vi "Set Value.vi"(8 "error in (no error)":errorcluster, 10 "Value":variant, 11 "IAttribute Data Type View in":refnum<class "IAttribute Data Type View.lvclass">) -> (0 "error out":errorcluster, 3 "IAttribute Data Type View out":refnum<class "IAttribute Data Type View.lvclass">)   [LabVIEW 2017, in "IAttribute Data Type View.lvclass"]
uses:
  <vilib>/gpm_packages/@cs/Test-executive-builder/Source/Test Executive Builder Dialogs/IAttribute Data Type View/IAttribute Data Type View.lvclass
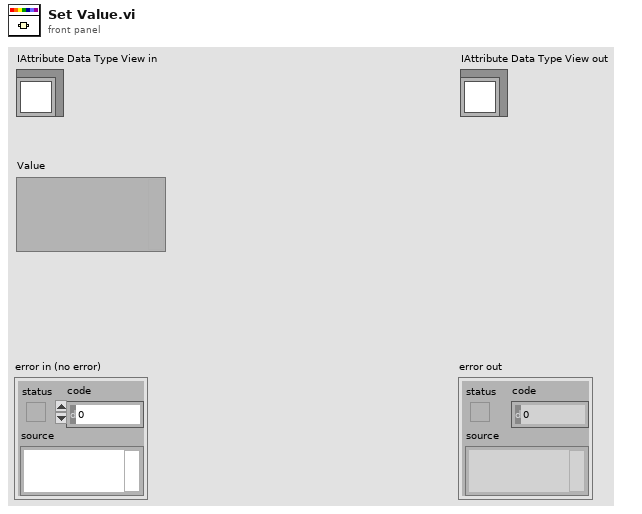
[diagram p1: front panel]
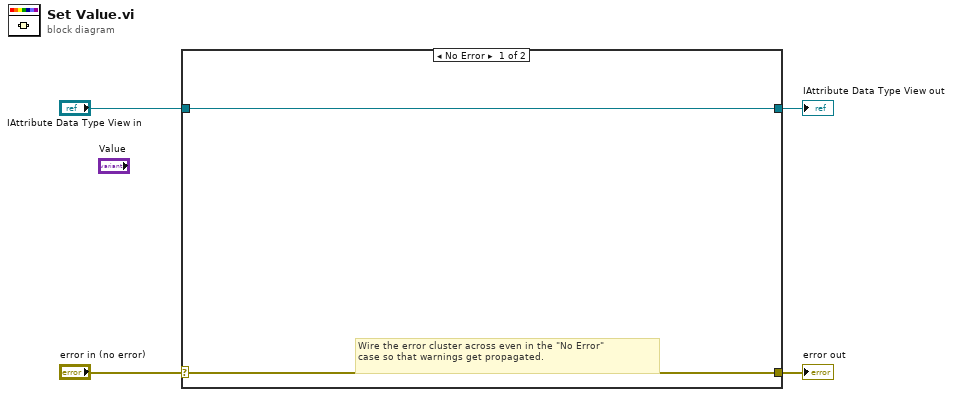
[diagram p0: block diagram]
diagram:
  n1 = case shown="No Error" "error in (no error)" {
    selector: "error in (no error)" -> [w5 w8]
    tunnel: [w5 w8] -> w3
    tunnel: [w6 w7] -> w1
    tunnel: "IAttribute Data Type View in" -> [w6 w7]
    frame No Error {
      # "Wire the error cluster across even in the \"No Error\"\ncase so that warnings get propagated."
    }
    frame Error {
    }
  }
  "error out" <- w3
  "IAttribute Data Type View out" <- w1
